vi "configure.vi"(8 "error in (no error)":errorcluster, 11 "LightSourceAN191011Chameleon in":refnum<class "LightSourceAN191011Chameleon.lvclass">) -> (0 "error out":errorcluster, 3 "LightSourceAN191011Chameleon out":refnum<class "LightSourceAN191011Chameleon.lvclass">)   [LabVIEW 2011, in "LightSourceAN191011Chameleon.lvclass"]
uses:
  LightSourceAN191011Chameleon.lvclass
  LightSourceAN191011Chameleon.lvclass/LightSourceAN191011Chameleon.ctl
  common/classes/GenericComponent/GenericComponent/GenericComponent.lvclass
panel:
  in  "start wavelength":dbl[unit]=6.800000000000001e-07 min=6.800000000000001e-07 max=1.08e-06 step=1e-09 format="%#_6f"
  in  "stop bits":u16=10
  in  "baud rate":u32
  in  "data bits":u16
  in  "parity":enum16{"None", "Odd", "Even", "Mark", "Space"}(ring)
  out "configuration":string
  in  "COM port":refnum<visa-resource-name>
  in  "delay before read":u32
  in  "cancel":bool
  in  "save":bool
  # "Configure AN191011Chameleon"
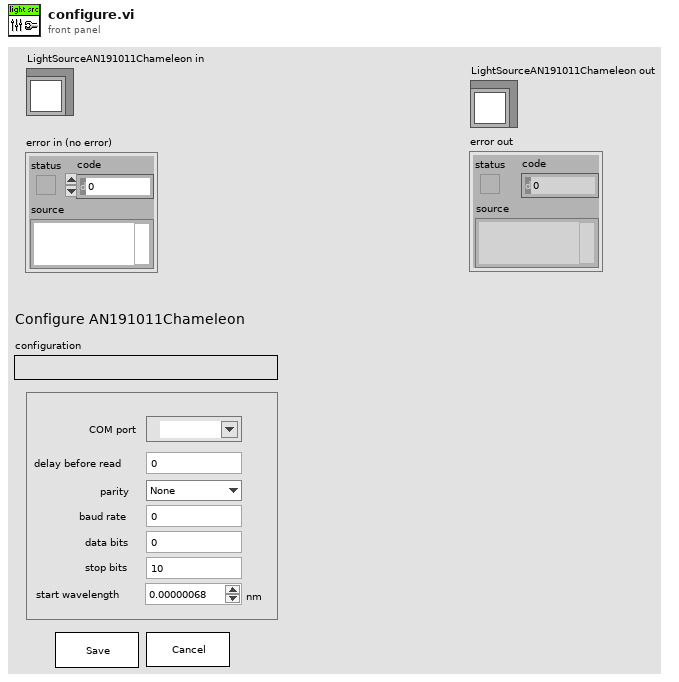
[diagram p1: front panel]
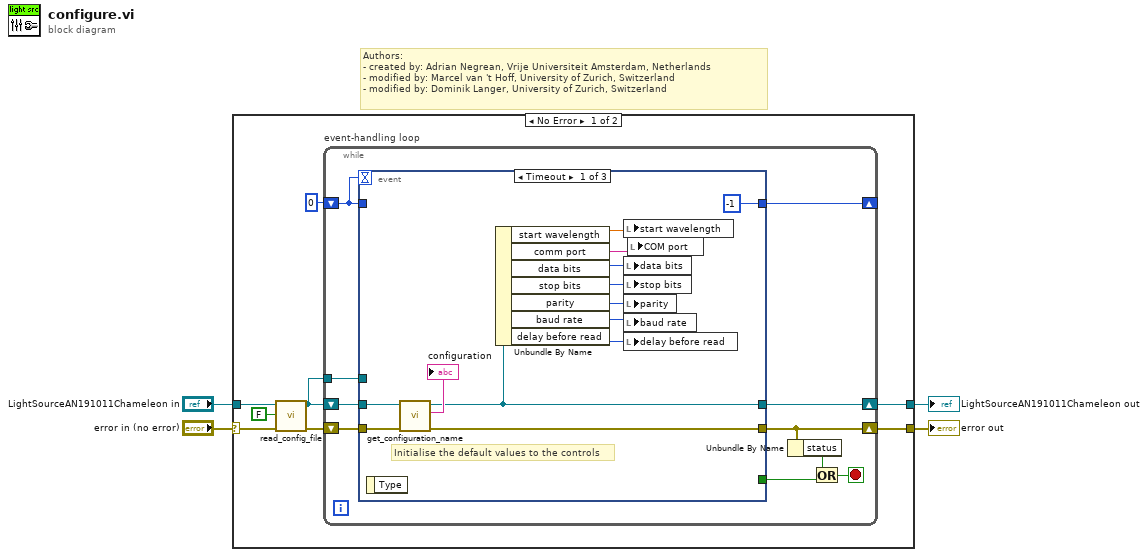
[diagram p0: block diagram]
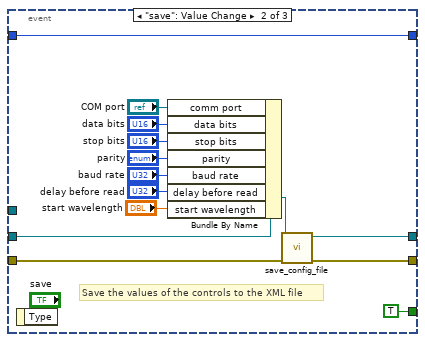
[diagram p2: hidden frame]
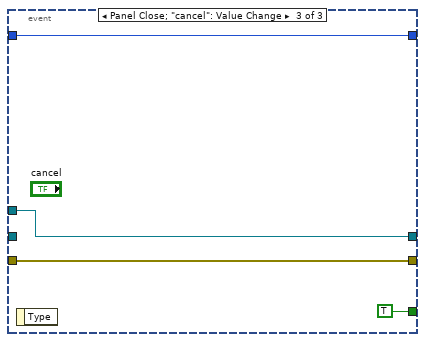
[diagram p3: hidden frame]
diagram:
  # "Authors: \n- created by: Adrian Negrean, Vrije Universiteit Amsterdam, Netherlands\n- modified by: Marcel van 't Hoff, University of Zurich, Switzerland\n- modified by: Dominik Langer, University of Zurich, Switzerland"
  n1 = case shown="No Error" "error in (no error)" {
    selector: "error in (no error)" -> [w10 w55]
    tunnel: [w7 w55] -> w3
    tunnel: [w6 w54] -> w1
    tunnel: "LightSourceAN191011Chameleon in" -> [w11 w54]
    frame No Error {
      n2 = call-dynamic "read_config_file.vi"("error in (no error)"=w10, "force load?"=FALSE, "GenericPlugin in"=w11) -> ("error out"=w9:errorcluster, "GenericPlugin out"=w5:refnum<class "LightSourceAN191011Chameleon.lvclass">)  [unwired: 7 in]
      n3 = while "event-handling loop" {
        shift-right: [w21] -> _
        shift-left: 0 -> [w22]
        shift-right: [w17] -> w6
        shift-left: w5 -> [w19]
        shift-right: [w14] -> w7
        shift-left: w9 -> [w18]
        tunnel: w5 -> [w13]
        stop <- w15 stop-if-true
        n4 = event shown="[0] Timeout" {
          selector: _ -> [_ _ _]
          dyn-events: _ -> [_ _ _]
          timeout: w22 -> [_ _ _]
          tunnel: w22 -> [_ w46 w51]
          tunnel: [-1 w46 w51] -> w21
          tunnel: w19 -> [w34 w36 _]
          tunnel: w18 -> [w33 w37 w53]
          tunnel: [w23 w49 w50] -> w17
          tunnel: [w24 w48 w53] -> w14
          tunnel: [_ TRUE TRUE] -> w16
          tunnel: w13 -> [_ _ w50]
          event Timeout {
            # "Initialise the default values to the controls"
            n5 = event-data() -> ()  [unwired: 1 in, 1 out]
            n6 = call "get_configuration_name.vi"("error in (no error)"=w33, "GenericPlugin.lvclass in"=w34) -> ("error out"=w24:errorcluster, "configuration name"=→"configuration":string, "GenericPlugin.lvclass out"=w23:refnum<class "LightSourceAN191011Chameleon.lvclass">)  [unwired: 7 in]
            n7 = Unbundle By Name(w23) -> ("start wavelength"=w25:dbl[unit], "comm port"=w32:string, "data bits"=w27:u16, "stop bits"=w28:u16, "parity"=w29:enum16{"None", "Odd", "Even", "Mark", "Space"}, "baud rate"=w26:u32, "delay before read"=w31:u32)
            n8 = local write "start wavelength"(w25) -> ()
            n9 = local write "data bits"(w27) -> ()
            n10 = local write "stop bits"(w28) -> ()
            n11 = local write "parity"(w29) -> ()
            n12 = local write "baud rate"(w26) -> ()
            n13 = local write "delay before read"(w31) -> ()
            n14 = local write "COM port"(w32) -> ()
          }
          event "save": Value Change {
            # "Save the values of the controls to the XML file"
            n15 = event-data() -> ()  [unwired: 1 in, 1 out]
            n16 = Bundle By Name(cluster=w36, "comm port"="COM port", "data bits"="data bits", "stop bits"="stop bits", "parity"="parity", "baud rate"="baud rate", "delay before read"="delay before read", "start wavelength"="start wavelength") -> (w45:refnum<class "LightSourceAN191011Chameleon.lvclass">)
            n17 = call-dynamic "save_config_file.vi"("error in (no error)"=w37, "GenericPlugin in"=w45) -> ("error out"=w48:errorcluster, "GenericPlugin out"=w49:refnum<class "LightSourceAN191011Chameleon.lvclass">)  [unwired: 8 in]
          }
          event Panel Close; "cancel": Value Change {
            n18 = event-data() -> ()  [unwired: 1 in, 1 out]
          }
        }
        n19 = Unbundle By Name(w14) -> ("status"=w20:bool)
        n20 = Or(x=w20, y=w16) -> (x .or. y?=w15:bool)
      }
    }
    frame Error {
    }
  }
  "error out" <- w3
  "LightSourceAN191011Chameleon out" <- w1
